vi "getDispCompVec.vi"(9 "Camera in":refnum<class "Camera.lvclass">, 10 "C3":dbl format="%#_13g", 11 "C2":dbl format="%#_13g") -> (3 "Gc":cdb[](array[numeric]))   [LabVIEW 2017]
uses:
  classes/HardwareObjects/Camera/Camera.lvclass
  classes/HardwareObjects/Camera/Camera.lvclass/Camera.ctl
  <vilib>/Analysis/1siggen.llb/Ramp Pattern by Samples.vi
  classes/HardwareObjects/Camera/Read Camera Dimensions.vi
  <vilib>/Analysis/NI_AALBase.lvlib
panel:
  out "k0":dbl
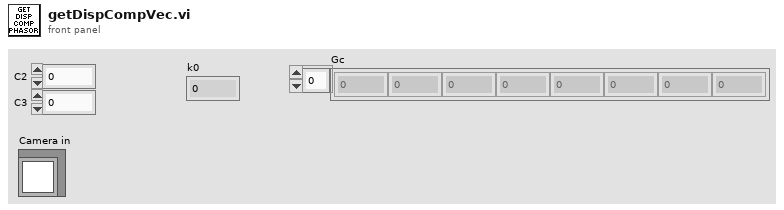
[diagram p1: front panel]
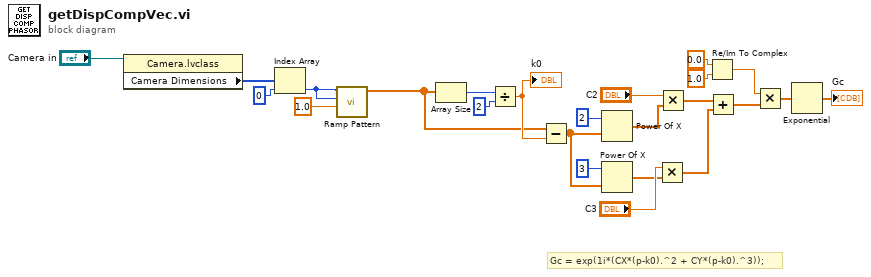
[diagram p0: block diagram]
diagram:
  # "Gc = exp(1i*(CX*(p-k0).^2 + CY*(p-k0).^3));"
  n1 = property class="Camera.lvclass"(reference="Camera in") -> ("Camera Dimensions"=w5:u16[])  [unwired: 1 in, 2 out]
  n2 = Index Array(array=w5, index=0) -> (element=w2:u16)
  n3 = call-poly <vilib>:"Ramp Pattern.vi"("start"=1.0, "end"=w2, "samples"=w2) -> ("Ramp Pattern"=w1:dbl[])  [unwired: 7 in, 1 out]
  n4 = Array Size(array=w1) -> (size(s)=w22:i32)
  n5 = Divide(x=w22, y=2) -> (x/y=w20:dbl)
  "k0" <- w20
  n6 = Subtract(x=w1, y=w20) -> (x-y=w17:dbl[])
  n7 = Power Of X(1:w17, 2:2 ("y")) -> (0:w15:dbl[])
  n8 = Power Of X(1:w17, 2:3 ("y")) -> (0:w13:dbl[])
  n9 = Multiply(x="C3", y=w13) -> (x*y=w11:dbl[])
  n10 = Multiply(x="C2", y=w15) -> (x*y=w12:dbl[])
  n11 = Re/Im To Complex(1:1.0 ("y"), 2:0.0 ("x")) -> (0:w9:cdb)
  n12 = Add(x=w12, y=w11) -> (x+y=w10:dbl[])
  n13 = Multiply(x=w9, y=w10) -> (x*y=w8:cdb[])
  n14 = Exponential(1:w8) -> (0:→"Gc":cdb[])
